vi "createNotInstance.vi"(8 "error in (no error)":errorcluster, 11 "reference in":refnum<class "Notification Controller.lvclass">) -> (0 "error out":errorcluster, 3 "reference out":refnum<class "Notification Controller.lvclass">)   [LabVIEW 2014, in "Notification Controller.lvclass"]
uses:
  Notification Controller.lvclass
  APP/itemsNotification_class/itemsNotification.lvclass
  APP/trackingNotification_class/trackingNotification.lvclass
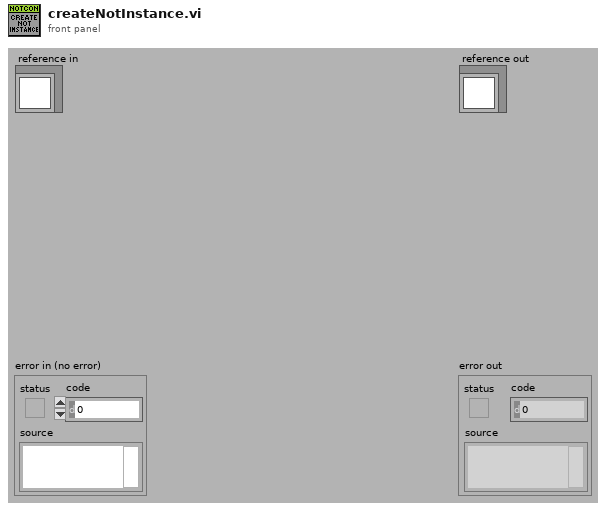
[diagram p1: front panel]
types:
  T1 = typedef "Notification Controller.lvclass/ObjectAttributesRef.ctl" = refnum<data-value>
  T2 = typedef "Notification Controller.lvclass/ObjectAttributes.ctl" = cluster{"MyAttribute":dbl, "items_data":string[][][], "items_notification_refs":refnum<class "itemsNotification.lvclass">[], "notifications_data_items":string[][], "items_nots?":bool, "devices_controller_ref":refnum<class "Devices Controller.lvclass">, "onlineUpdate":timestamp, "notController?":bool, "tracking_notification_ref":refnum<class "trackingNotification.lvclass">, "notifications_data_tracking":string[][], "tracking_parts_data":string[][], "tracking_nots?":bool, "index_tracking_not":i32[], "file_controller_ref":refnum<class "File Controller.lvclass">}
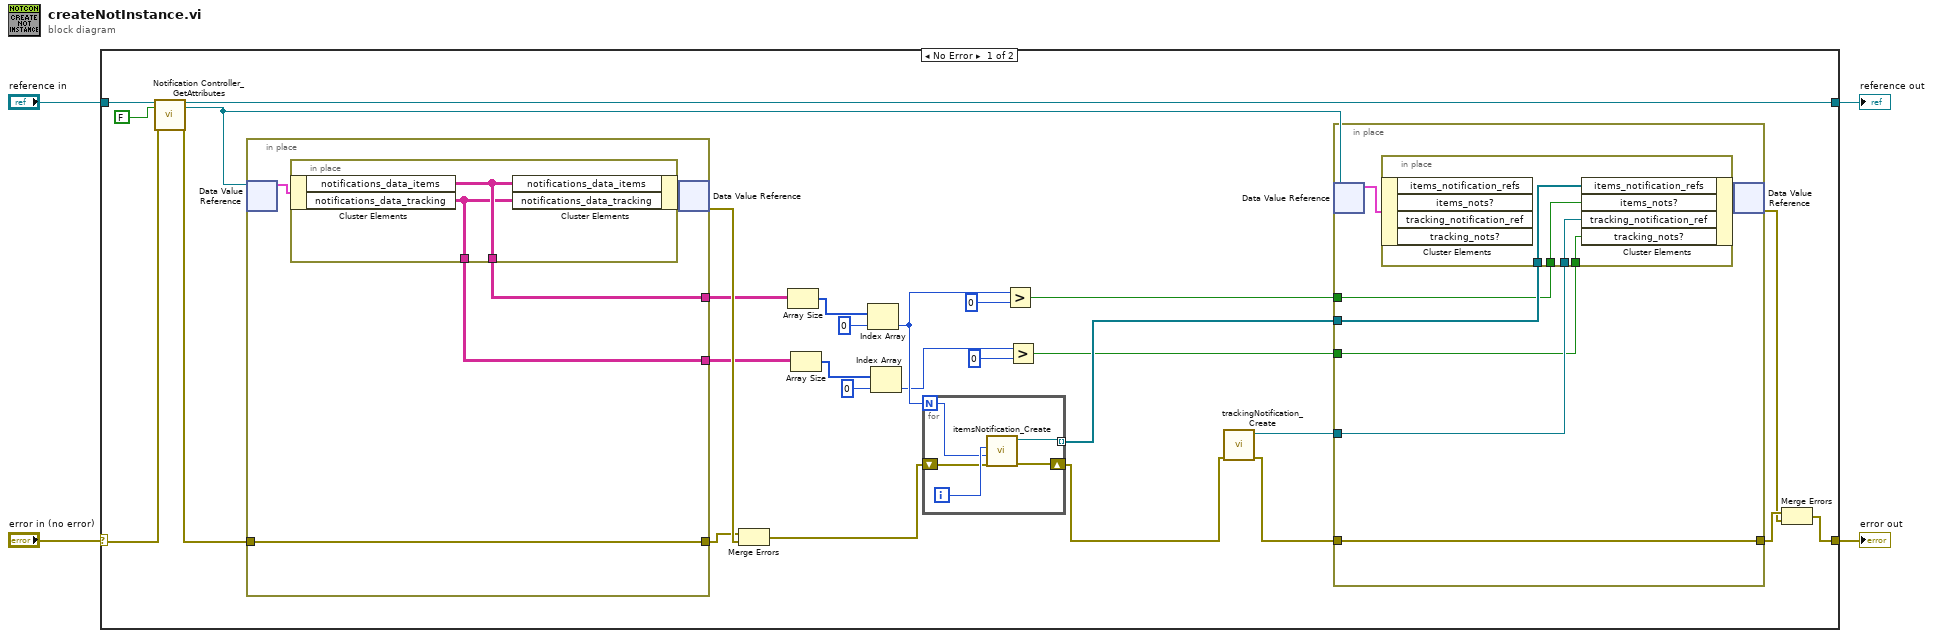
[diagram p0: block diagram]
diagram:
  n1 = case shown="No Error" "error in (no error)" {
    selector: "error in (no error)" -> [w28 w57]
    tunnel: [w22 w57] -> w3
    tunnel: [w26 w56] -> w1
    tunnel: "reference in" -> [w30 w56]
    frame No Error {
      n2 = call "Notification Controller_GetAttributes.vi"("reference in"=w30, "return data? (T)"=FALSE, "error in (no error)"=w28) -> ("reference out"=w26:refnum<class "Notification Controller.lvclass">, "attributes ref"=w21:T1, "error out"=w27:errorcluster)  [unwired: 13 in, 1 out]
      n3 = in-place {
        in-place-border: w27 -> [w51]
        in-place-border: [w51] -> w31
        in-place-border: [w50] -> w19
        in-place-border: [w49] -> w9
        n4 = in-place-dvr #1(w21) -> (w52:T2)  [unwired: 1 out]
        n5 = in-place {
          in-place-border: [w55] -> w50
          in-place-border: [w54] -> w49
          n6 = in-place-cluster #2(w52) -> ("notifications_data_items"=w55:string[][], "notifications_data_tracking"=w54:string[][])
          n7 = in-place-cluster #2("notifications_data_items"=w55, "notifications_data_tracking"=w54) -> (w53:T2)
        }
        n8 = in-place-dvr #1(w53) -> (w32:errorcluster)  [unwired: 1 out]
      }
      n9 = Merge Errors(w31, w32) -> (w25:errorcluster)
      n10 = Array Size(array=w19) -> (size(s)=w18:i32[])
      n11 = Array Size(array=w9) -> (size(s)=w10:i32[])
      n12 = Index Array(array=w18, index=0) -> (element=w16:i32)
      n13 = Index Array(array=w10, index=0) -> (element=w12:i32)
      n14 = for {
        N: w16 -> [w45]
        shift-right: [w47] -> w8
        shift-left: w25 -> [w46]
        tunnel: [w44] -> w20 mode=indexing
        i -> [w48]
        n15 = call "itemsNotification_Create.vi"("error in (no error)"=w46, "dim"=w45, "index"=w48) -> ("error out"=w47:errorcluster, "reference out"=w44:refnum<class "itemsNotification.lvclass">)  [unwired: 7 in]
      }
      n16 = Greater?(x=w16, y=0) -> (0:w14:bool)
      n17 = Greater?(x=w12, y=0) -> (0:w5:bool)
      n18 = call "trackingNotification_Create.vi"("error in (no error)"=w8) -> ("error out"=w7:errorcluster, "reference out"=w6:refnum<class "trackingNotification.lvclass">)  [unwired: 9 in]
      n19 = in-place {
        in-place-border: w7 -> [w37]
        in-place-border: [w37] -> w24
        in-place-border: w20 -> [w36]
        in-place-border: w14 -> [w35]
        in-place-border: w6 -> [w34]
        in-place-border: w5 -> [w33]
        n20 = in-place-dvr #3(w21) -> (w38:T2)  [unwired: 1 out]
        n21 = in-place {
          in-place-border: w36 -> [w43]
          in-place-border: w35 -> [w42]
          in-place-border: w34 -> [w41]
          in-place-border: w33 -> [w40]
          n22 = in-place-cluster #4(w38) -> ()  [unwired: 4 out]
          n23 = in-place-cluster #4("items_notification_refs"=w43, "items_nots?"=w42, "tracking_notification_ref"=w41, "tracking_nots?"=w40) -> (w39:T2)
        }
        n24 = in-place-dvr #3(w39) -> (w23:errorcluster)  [unwired: 1 out]
      }
      n25 = Merge Errors(w24, w23) -> (w22:errorcluster)
    }
    frame Error {
    }
  }
  "error out" <- w3
  "reference out" <- w1
